vi "Out_S5F1.vi"(8 "error in (no error)":errorcluster, 10 "S5F1":T1, 11 "S5 Message Class in":refnum<class "S5 Message Class.lvclass">) -> (0 "error out":errorcluster, 3 "S5 Message Class out":refnum<class "S5 Message Class.lvclass">)   [LabVIEW 2020, in "SECS Communication.lvlib" / "S5 Message Class.lvclass"]
uses:
  S5 Message Class.lvclass
  D:/Dropbox/SECS/SECS_GEM v1.0.6/Com/SECS Communication/SECS-II Class/SECS-II Class.lvclass
  S5F1.ctl
  SECS-II Class/Data Message_List.vi
  SECS-II Class/Data Message_Binary.vi
  SECS-II Class/Data Message_U4.vi
  SECS-II Class/Data Message_ASCII.vi
  SECS-II Class/SECS-II Class.lvclass
  D:/Dropbox/SECS/SECS_GEM v1.0.6/Com/SECS Communication/S5 Message Class/S5 Message Class.lvclass
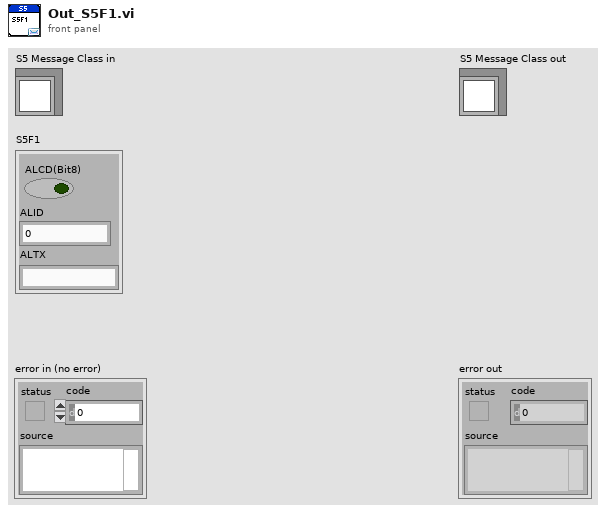
[diagram p1: front panel]
types:
  T1 = typedef "SECS Communication.lvlib/S5 Message Class.lvclass/S5F1.ctl" = cluster{"ALCD(Bit8)":bool, "ALID":u32, "ALTX":string}
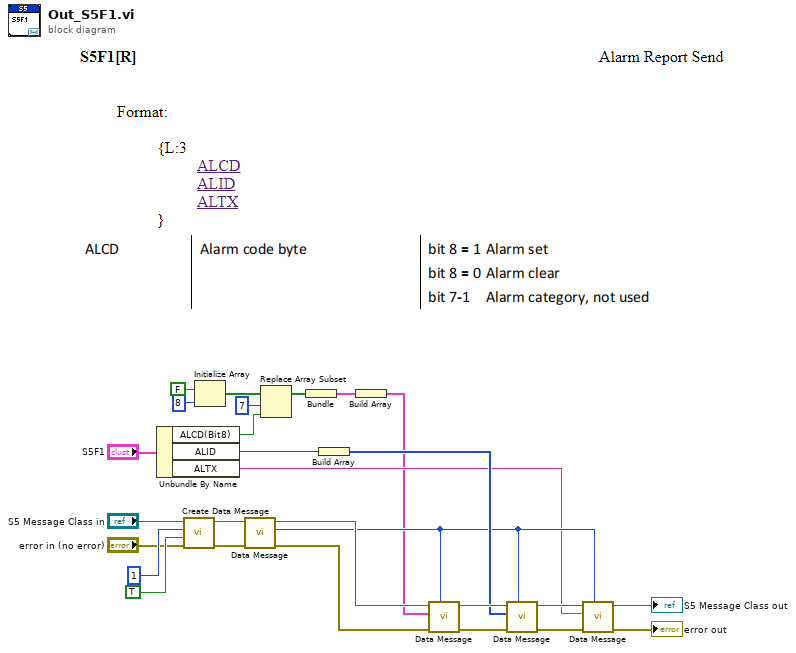
[diagram p0: block diagram]
diagram:
  n1 = Unbundle By Name("S5F1") -> ("ALCD(Bit8)"=w5:bool, "ALID"=w16:u32, "ALTX"=w11:string)
  n2 = call "Create Data Message.vi"("error in (no error)"="error in (no error)", "W-Bit"=TRUE, "Function"=u8 1, "SECS-II Class in"="S5 Message Class in") -> ("error out"=w24:errorcluster, "SECS-II Class out"=w25:refnum<class "S5 Message Class.lvclass">)  [unwired: 6 in]
  n3 = Initialize Array(FALSE, 8 ("dimension size")) -> (w6:bool[])
  n4 = call-poly "Data Message.vi"("error in"=w24, "SECS-II Class in"=w25) -> ("error out"=w21:errorcluster, "Index"=w13:i32, "SECS-II Class out"=w20:refnum<class "S5 Message Class.lvclass">)  [unwired: 7 in]
  n5 = Replace Array Subset(array=w6, new element=w5, index=7) -> (w3:bool[])
  n6 = Bundle(w3) -> (w2:cluster{bool[]})  [unwired: 1 in]
  n7 = Build Array(w16) -> (w15:u32[])
  n8 = Build Array(w2) -> (w1:cluster{bool[]}[])
  n9 = call-poly "Data Message.vi"("Parent Index"=w13, "error in"=w21, "Data Cluster"=w1, "SECS-II Class in"=w20) -> ("error out"=w17:errorcluster, "SECS-II Class out"=w18:refnum<class "S5 Message Class.lvclass">)  [unwired: 6 in]
  n10 = call-poly "Data Message.vi"("Parent Index"=w13, "error in"=w17, "Data"=w15, "SECS-II Class in"=w18) -> ("error out"=w12:errorcluster, "SECS-II Class out"=w14:refnum<class "S5 Message Class.lvclass">)  [unwired: 6 in]
  n11 = call-poly "Data Message.vi"("Parent Index"=w13, "error in"=w12, "Data"=w11, "SECS-II Class in"=w14) -> ("error out"=→"error out":errorcluster, "SECS-II Class out"=→"S5 Message Class out":refnum<class "S5 Message Class.lvclass">)  [unwired: 6 in]
